vi "temp_conv.vi"() -> ()   [LabVIEW 2023]
uses:
  <vilib>/express/express arith-compare/Formula/XNode/ExpressFormulaBlockNode.xnode
panel:
  out "K":dbl(slide) scale=233.0..450.0
  out "F":dbl(slide) scale=-40.0..300.0
  out "KELVIN":dbl
  out "FAHRENHEIT":dbl
  in  "CELSIUS":dbl
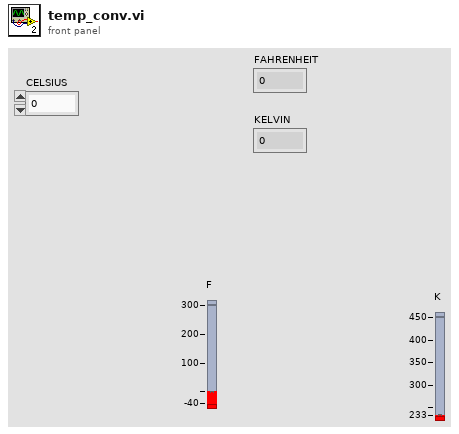
[diagram p1: front panel]
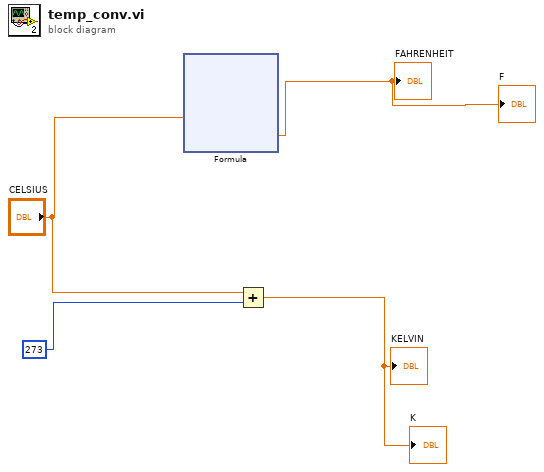
[diagram p0: block diagram]
diagram:
  n1 = xnode "Formula"("X1"="CELSIUS") -> ("Result"=→"FAHRENHEIT" →"F":dbl)  [unwired: 1 in, 1 out]
  n2 = Add(x="CELSIUS", y=273) -> (x+y=→"KELVIN" →"K":dbl)
